vi "2-2-2 Format Into String.vi"() -> ()   [LabVIEW 2020]
panel:
  out "JSON String":string
  in  "motor_on":bool
  in  "pressure":dbl=1.013
  in  "temperature":dbl=82.3
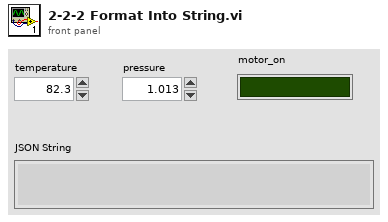
[diagram p1: front panel]
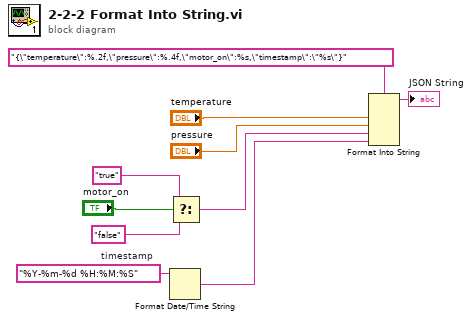
[diagram p0: block diagram]
diagram:
  w7 = "%Y-%m-%d %H:%M:%S"  # timestamp
  n1 = Format Date/Time String(time format string (%c)=w7) -> (date/time string=w8:string)  [unwired: 2 in]
  n2 = Select(t="true" ("timestamp"), s="motor_on", f="false" ("timestamp")) -> (s? t:f=w2:string)
  n3 = Format Into String(format string="{\"temperature\":%.2f,\"pressure\":%.4f,\"motor_on\":%s,\"timestamp\":\"%s\"}", "temperature", "pressure", w2, w8) -> (resulting string=→"JSON String":string)  [unwired: 2 in, 1 out]
